vi "Measurement-SP.vi"(1 "Ctl Refnum 2":refnum<vi>, 2 "Ctl Refnum":refnum<vi>, 5 "时间间隔":dbl=2.0, 7 "Scanning Mode":u16(ring)=1 items=["Linear", "Log"], 8 "error in (no error)":errorcluster, 9 "Byte Stream File Refnum":refnum<file>, 10 "客户仪器地址":refnum<visa-resource-name>="USB0::0x0471::0x2826::QF71600867::INSTR", 11 "开始频率":dbl[](array[numeric])=[20.0, 5000000.0, 100.0]) -> (0 "error out":errorcluster, 4 "Array":string[][](array[string]))   [LabVIEW 2017]
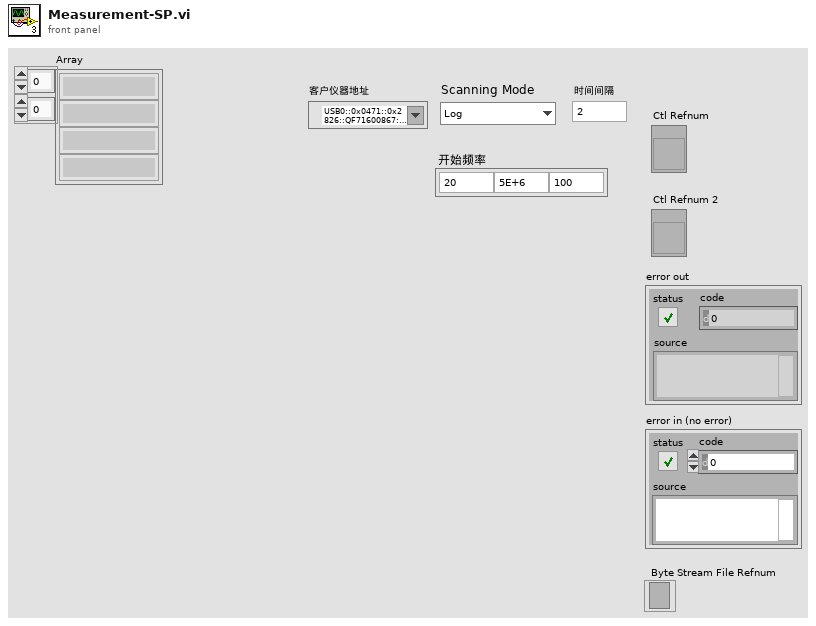
[diagram p1: front panel]
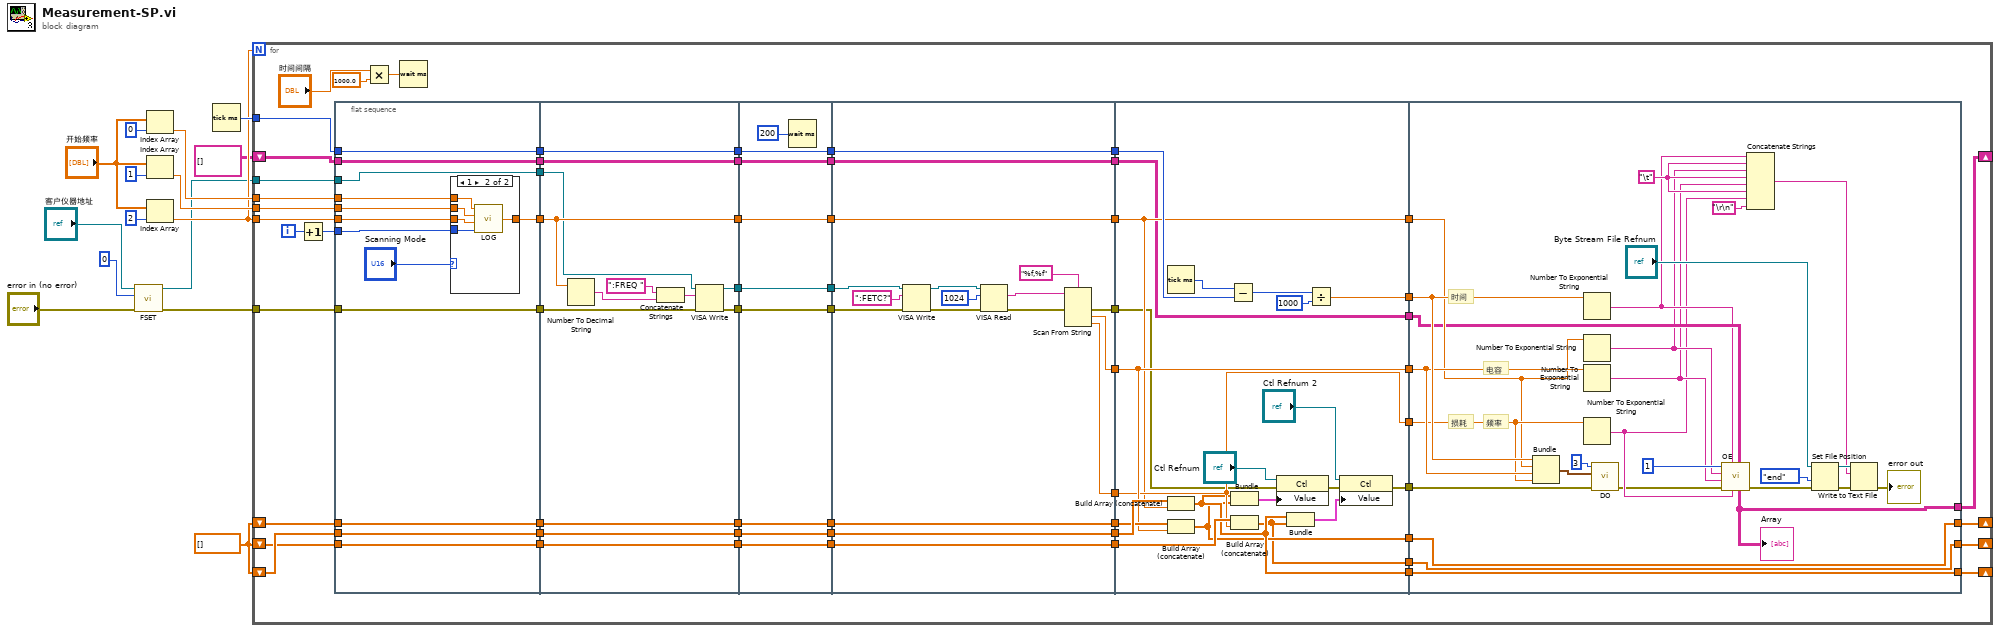
[diagram p0: block diagram]
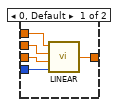
[diagram p2: hidden frame]
diagram:
  w10 = dbl[] []
  n1 = call "FSET.vi"("error in (no error)"="error in (no error)", "Function (0: Cp-D)"=0, "VISA resource name"="客户仪器地址") -> ("error out"=w2:errorcluster, "VISA resource name out"=w1:refnum<visa-resource-name>)  [unwired: 7 in]
  n2 = Index Array(array="开始频率", index=0 ("索引")) -> (element=w9:dbl)
  n3 = Index Array(array="开始频率", index=1 ("索引")) -> (element=w8:dbl)
  n4 = Index Array(array="开始频率", index=2 ("索引")) -> (element=w7:dbl)
  n5 = Tick Count (ms)() -> (millisecond timer value=w11:u32)
  n6 = for {
    N: w7 -> [_]
    tunnel: w7 -> [w74]
    tunnel: w9 -> [w73]
    tunnel: w8 -> [w72]
    tunnel: w11 -> [w71]
    shift-right: [w69] -> _
    shift-left: w10 -> [w70]
    shift-right: [w67] -> _
    shift-left: w10 -> [w68]
    shift-right: [w66] -> _
    shift-left: w10 -> [w65]
    shift-right: [w22] -> _
    shift-left: string[][] [] -> [w61]
    tunnel: w2 -> [w19]
    tunnel: w1 -> [w17]
    i -> [w76]
    n7 = Increment(x=w76) -> (x+1=w75:i32)
    n8 = flat-sequence {
      tunnel: w75 -> [w89]
      tunnel: w74 -> [w88]
      tunnel: w73 -> [w87]
      tunnel: w72 -> [w86]
      tunnel: w71 -> [w83]
      tunnel: w70 -> [w82]
      tunnel: w68 -> [w81]
      tunnel: w65 -> [w80]
      tunnel: w61 -> [w79]
      tunnel: [w83] -> w60
      tunnel: [w82] -> w59
      tunnel: [w81] -> w58
      tunnel: [w80] -> w57
      tunnel: [w85] -> w56
      tunnel: [w79] -> w55
      tunnel: w19 -> [w77]
      tunnel: [w78] -> w18
      tunnel: w17 -> [w78]
      tunnel: [w77] -> w16
      tunnel: w60 -> [w108]
      tunnel: w59 -> [w107]
      tunnel: w58 -> [w106]
      tunnel: w57 -> [w105]
      tunnel: w56 -> [w110]
      tunnel: w55 -> [w104]
      tunnel: [w108] -> w54
      tunnel: [w107] -> w53
      tunnel: [w106] -> w52
      tunnel: [w105] -> w51
      tunnel: [w110] -> w50
      tunnel: [w102] -> w49
      tunnel: [w104] -> w48
      tunnel: [w103] -> w20
      tunnel: w18 -> [w101]
      tunnel: w16 -> [w100]
      tunnel: w54 -> [w120]
      tunnel: w53 -> [w119]
      tunnel: w52 -> [w118]
      tunnel: w51 -> [w117]
      tunnel: w50 -> [w116]
      tunnel: w49 -> [w115]
      tunnel: w48 -> [w114]
      tunnel: [w120] -> w47
      tunnel: [w119] -> w46
      tunnel: [w118] -> w45
      tunnel: [w117] -> w44
      tunnel: [w116] -> w43
      tunnel: [w115] -> w42
      tunnel: [w114] -> w41
      tunnel: [w113] -> w21
      tunnel: w20 -> [w113]
      tunnel: w47 -> [w128]
      tunnel: w46 -> [w127]
      tunnel: w45 -> [w126]
      tunnel: w44 -> [w125]
      tunnel: w43 -> [w124]
      tunnel: w42 -> [w131]
      tunnel: w41 -> [w123]
      tunnel: [w128] -> w40
      tunnel: [w127] -> w39
      tunnel: [w126] -> w38
      tunnel: [w125] -> w37
      tunnel: [w124] -> w36
      tunnel: [w133] -> w35
      tunnel: [w132] -> w34
      tunnel: [w129] -> w33
      tunnel: [w123] -> w32
      tunnel: w21 -> [w122]
      tunnel: w40 -> [w160]
      tunnel: w39 -> [w157]
      tunnel: w38 -> [w156]
      tunnel: w37 -> [w154]
      tunnel: w36 -> [w148]
      tunnel: w35 -> [w155]
      tunnel: w34 -> [w153]
      tunnel: w33 -> [w142]
      tunnel: w32 -> [w147]
      tunnel: [w152] -> w31
      tunnel: [w151] -> w30
      tunnel: [w150] -> w29
      tunnel: [w148] -> w28
      tunnel: [w155] -> w27
      tunnel: [w153] -> w26
      tunnel: [w149] -> w25
      tunnel: [w143] -> w24
      tunnel: [w147] -> w23
      tunnel: [w165] -> w69
      tunnel: [w164] -> w67
      tunnel: [w163] -> w66
      tunnel: [w162] -> w22
      tunnel: w31 -> [w165]
      tunnel: w30 -> [w164]
      tunnel: w29 -> [w163]
      tunnel: w28 -> [w177]
      tunnel: w27 -> [w179]
      tunnel: w26 -> [w178]
      tunnel: w25 -> [w180]
      tunnel: w24 -> [w167]
      tunnel: w23 -> [w175]
      frame #0 {
        n9 = case shown="1" "Scanning Mode" {
          tunnel: w89 -> [w94 w99]
          tunnel: w88 -> [w93 w98]
          tunnel: w87 -> [w92 w97]
          tunnel: w86 -> [w91 w96]
          tunnel: [w90 w95] -> w85
          frame 0, Default {
            n10 = call "LINEAR.vi"("I"=w94, "N"=w93, "END"=w91, "INITIAL"=w92) -> ("数值"=w90:dbl)
          }
          frame 1 {
            n11 = call "LOG.vi"("I"=w99, "N"=w98, "END"=w96, "INITIAL"=w97) -> ("数值"=w95:dbl)
          }
        }
      }
      frame #1 {
        n12 = Number To Decimal String(number=w110) -> (decimal integer string=w111:string)  [unwired: 1 in]
        n13 = Concatenate Strings(":FREQ " ("字符串"), w111) -> (w109:string)
        n14 = VISA Write(VISA resource name=w101, write buffer=w109, error in (no error)=w100) -> (VISA resource name out=w103:refnum<visa-resource-name>, error out=w102:errorcluster)  [unwired: 1 out]
      }
      frame #2 {
        n15 = Wait (ms)(milliseconds to wait=u32 200 ("等待时间（毫秒）")) -> ()  [unwired: 1 out]
      }
      frame #3 {
        n16 = VISA Write(VISA resource name=w122, write buffer=":FETC?" ("写入缓冲区"), error in (no error)=w131) -> (VISA resource name out=w137:refnum<visa-resource-name>, error out=w138:errorcluster)  [unwired: 1 out]
        n17 = VISA Read(VISA resource name=w137, byte count=u32 1024 ("字节总数"), error in (no error)=w138) -> (read buffer=w135:string, error out=w130:errorcluster)  [unwired: 2 out]
        n18 = Scan From String(format string="%f,%f" ("格式字符串"), input string=w135, error in=w130) -> (error out=w129:errorcluster, output 1=w133:dbl, output 2=w132:dbl)  [unwired: 3 in, 2 out]
      }
      frame #4 {
        n19 = Tick Count (ms)() -> (millisecond timer value=w161:u32)
        n20 = Build Array (concatenate)(w157, w148) -> (w152:dbl[])
        n21 = Build Array (concatenate)(w156, w155) -> (w151:dbl[])
        n22 = Subtract(x=w161, y=w160) -> (x-y=w159:u32)
        n23 = Bundle(w152, w151) -> (w141:cluster{dbl[], dbl[]})  [unwired: 1 in]
        n24 = Build Array (concatenate)(w154, w153) -> (w150:dbl[])
        n25 = property class="Ctl"(reference="Ctl Refnum", error in=w142, "Value"=w141) -> (error out=w144:errorcluster)  [unwired: 1 out]
        n26 = Bundle(w152, w150) -> (w140:cluster{dbl[], dbl[]})  [unwired: 1 in]
        n27 = Divide(x=w159, y=u32 1000) -> (x/y=w149:dbl)
        n28 = property class="Ctl"(reference="Ctl Refnum 2", error in=w144, "Value"=w140) -> (error out=w143:errorcluster)  [unwired: 1 out]
      }
      frame #5 {
        w184 = "\t"
        # "损耗"
        # "电容"
        # "频率"
        # "时间"
        n29 = Bundle(w180, "数值"=w177, w179, w178) -> (w168:cluster{dbl, "数值":dbl, dbl, dbl})  [unwired: 1 in]
        n30 = Number To Exponential String(number=w180) -> (E-format string=w174:string)  [unwired: 3 out]
        n31 = Number To Exponential String(number=w177) -> (E-format string=w173:string)  [unwired: 3 out]
        n32 = Number To Exponential String(number=w179) -> (E-format string=w172:string)  [unwired: 3 out]
        n33 = Number To Exponential String(number=w178) -> (E-format string=w171:string)  [unwired: 3 out]
        n34 = call "DO.vi"("error in (no error)"=w167, "数据输出"=w168, "功能编号"=3) -> ("error out"=w166:errorcluster)  [unwired: 8 in]
        n35 = call "OE.vi"("Array"=w175, "String 4"=w171, "String"=w174, "error in (no error)"=w166, "String 3"=w172, "String 2"=w173, "Numeric"=1) -> ("error out"=w170:errorcluster, "Array 2"=w162:string[][])  [unwired: 2 in, 1 out]
        "Array" <- w162
        n36 = Concatenate Strings(w174, w184, w173, w184, w172, w184, w171, "\r\n") -> (w186:string)
        n37 = Set File Position(refnum="Byte Stream File Refnum", from (0:start)=enum16{"start", "end", "current"}."end" ("自（0:起始）"), error in=w170) -> (refnum out=w188:refnum<file>, error out=w185:errorcluster)  [unwired: 1 out]
        n38 = Write to Text File(file (use dialog)=w188, text=w186, error in=w185) -> (error out=→"error out":errorcluster)  [unwired: 3 out]
      }
    }
    n39 = Multiply(x="时间间隔", y=1000.0) -> (x*y=w62:dbl)
    n40 = Wait (ms)(milliseconds to wait=w62) -> ()  [unwired: 1 out]
  }
